vi "Send Reply Msg DataSocket.vi"(6 "Reply Protocol DataSocket in":refnum<class "Reply Protocol DataSocket.lvclass">, 7 "Message Priority (Normal)":T1=enum."Normal", 8 "error in":errorcluster, 11 "Message Enqueuer":refnum<class "Message Enqueuer.lvclass">) -> (0 "error out":errorcluster, 1 "Timeout?":bool, 2 "Reply":variant, 3 "Message Enqueuer out":refnum<class "Message Enqueuer.lvclass">)   [LabVIEW 2023, in "Target Reply Time Test Actor.lvlib" / "Reply Msg DataSocket Msg.lvclass"]
doc: "This VI sends the message to an actor."
uses:
  Reply Msg DataSocket Msg.lvclass
  Reply Msg DataSocket Msg.lvclass/Reply Msg DataSocket Msg.ctl
  Reply Msg DS/Reply Msg DataSocket.lvclass
  D:/git/Reply-Msg-DataSocket/Reply Msg DS/Reply Msg DataSocket.lvclass
  C:/Program Files/National Instruments/LabVIEW 2023/vi.lib/ActorFramework/Message/Message.lvclass
  D:/git/Reply-Msg-DataSocket/Tests/Target Reply Time Test Actor/Target Reply Time Test Actor Messages/Reply Msg DataSocket Msg/Reply Msg DataSocket Msg.lvclass
  <vilib>/ActorFramework/Message Enqueuer/Message Enqueuer.lvclass
  <vilib>/ActorFramework/Message Enqueuer/Message Priority.ctl
  HAL/HAL GOOP4/Reply Protocol/Reply Protocol DataSocket/Reply Protocol DataSocket.lvclass
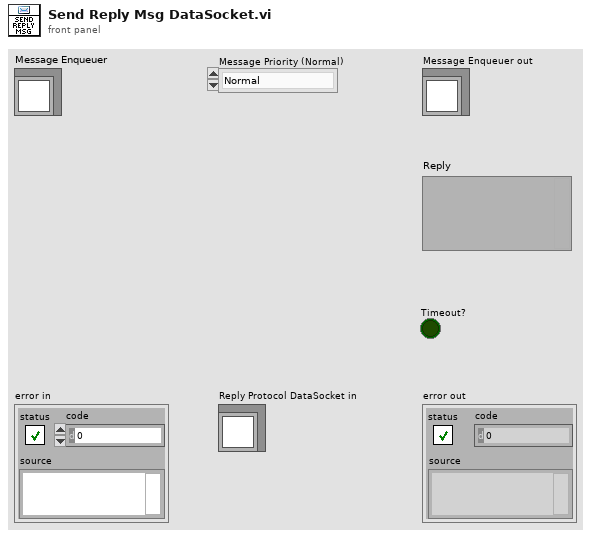
[diagram p1: front panel]
types:
  T1 = typedef "Actor Framework.lvlib/Message Enqueuer.lvclass/Message Priority.ctl" = enum16{"Low", "Normal", "High"}
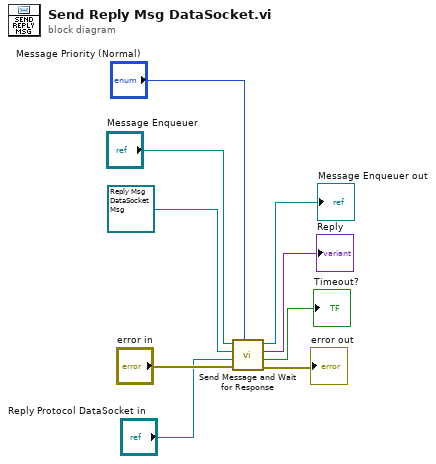
[diagram p0: block diagram]
diagram:
  n1 = call "Send Message and Wait for Response.vi"("Message Priority (Normal)"="Message Priority (Normal)", "error in"="error in", "Reply Protocol DataSocket in"="Reply Protocol DataSocket in", "Original Message"=refnum<class "Reply Msg DataSocket Msg.lvclass"> refnum ("Target Reply Time Test Actor.lvlib:Reply Msg DataSocket Msg.lvclass"), "Message Enqueuer in"="Message Enqueuer") -> ("error out"=→"error out":errorcluster, "Timeout?"=→"Timeout?":bool, "Reply"=→"Reply":variant, "Message Enqueuer out"=→"Message Enqueuer out":refnum<class "Message Enqueuer.lvclass">)  [unwired: 3 in]
